vi "alignObjects.vi"(6 "alignment":T1, 8 "error in (no error)":errorcluster, 11 "GObjectsIn":refnum<class "GObject.lvclass">[](array[class])) -> (0 "error out":errorcluster, 3 "GObjectsOut":refnum<class "GObject.lvclass">[](array[class]))   [LabVIEW 2023, in "TLC_Scripto.lvlib"]
uses:
  TLC_Scripto.lvlib
  GObject/GObject.lvclass
  Ctrls/alignment.ctl
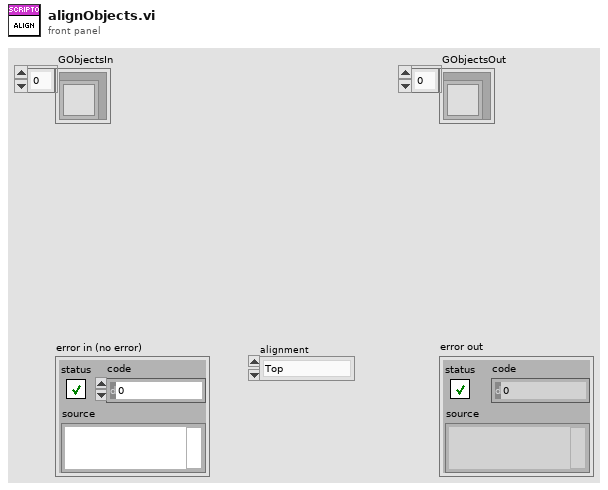
[diagram p1: front panel]
types:
  T1 = typedef "TLC_Scripto.lvlib/alignment.ctl" = enum16{"Top", "Bottom", "Left", "Right", "Center"}
  T2 = typedef "TLC_Scripto.lvlib/rectangle.ctl" = cluster{"left":i32, "top":i32, "right":i32, "bottom":i32}
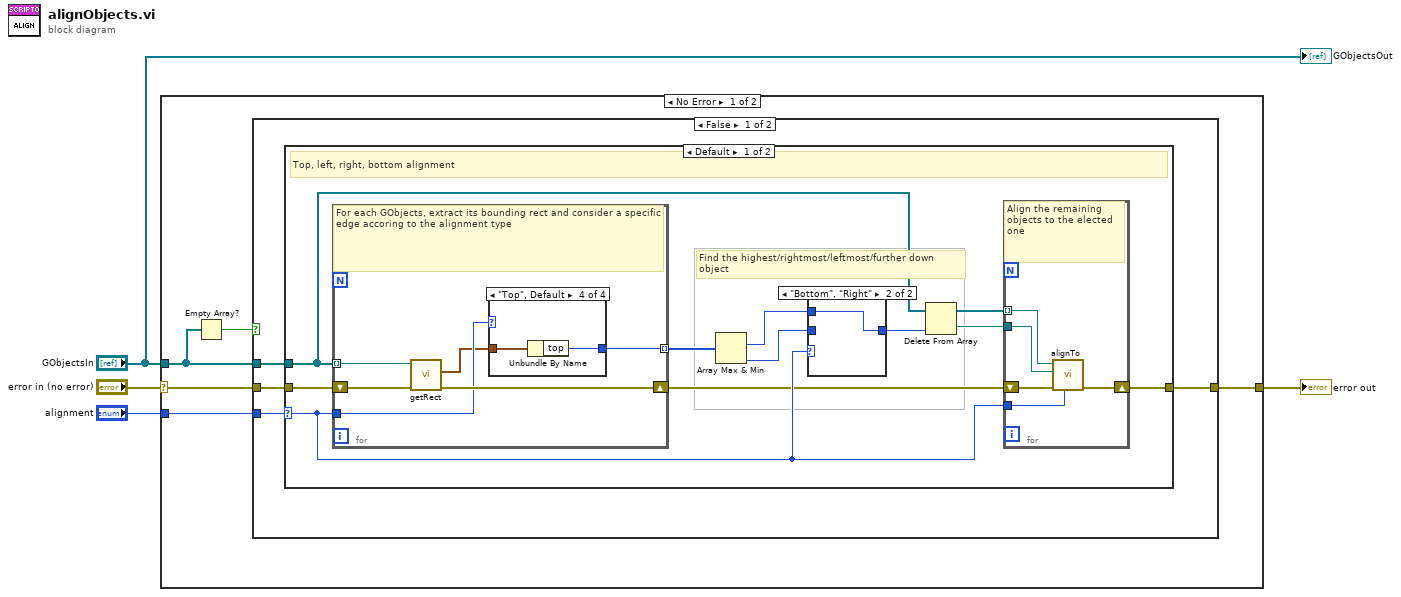
[diagram p0: block diagram]
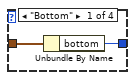
[diagram p3: hidden frame]
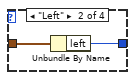
[diagram p4: hidden frame]
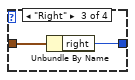
[diagram p5: hidden frame]
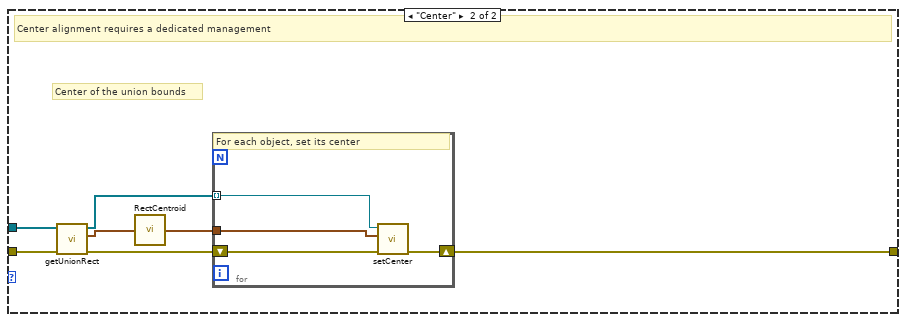
[diagram p6: hidden frame]
diagram:
  n1 = case shown="No Error" "error in (no error)" {
    selector: "error in (no error)" -> [w9 w58]
    tunnel: "GObjectsIn" -> [w7 _]
    tunnel: [w8 w58] -> w3
    tunnel: "alignment" -> [w5 _]
    frame No Error {
      n2 = Empty Array?(array=w7) -> (empty?=w6:bool)
      n3 = case shown="False" w6 {
        tunnel: w9 -> [w11 w57]
        tunnel: [w13 w57] -> w8
        tunnel: w7 -> [w12 _]
        tunnel: w5 -> [w10 _]
        frame False {
          n4 = case shown="Default" w10 {
            selector: w10 -> [w16 _]
            tunnel: [w14 w52] -> w13
            tunnel: w12 -> [w20 w50]
            tunnel: w11 -> [w24 w48]
            frame Default {
              # "Find the highest/rightmost/leftmost/further down object"
              # "Top, left, right, bottom alignment"
              n5 = for {
                tunnel: w20 -> [w37] mode=indexing
                shift-right: [w35] -> w15
                shift-left: w24 -> [w36]
                tunnel: w16 -> [w34]
                tunnel: [w32] -> w23 mode=indexing
                # "For each GObjects, extract its bounding rect and consider a specific edge accoring to the alignment type"
                n6 = call-dynamic "getRect.vi"("error in (no error)"=w36, "GObject in"=w37) -> ("error out"=w35:errorcluster, "rectangle"=w33:T2)  [unwired: 7 in, 1 out]
                n7 = case shown="\"Top\", Default" w34 {
                  tunnel: w33 -> [w39 w41 w43 w45]
                  tunnel: [w38 w40 w42 w44] -> w32
                  frame "Bottom" {
                    n8 = Unbundle By Name(w39) -> ("bottom"=w38:i32)
                  }
                  frame "Left" {
                    n9 = Unbundle By Name(w41) -> ("left"=w40:i32)
                  }
                  frame "Right" {
                    n10 = Unbundle By Name(w43) -> ("right"=w42:i32)
                  }
                  frame "Top", Default {
                    n11 = Unbundle By Name(w45) -> ("top"=w44:i32)
                  }
                }
              }
              n12 = Array Max & Min(array=w23) -> (max index (indices)=w21:i32, min index (indices)=w22:i32)  [unwired: 2 out]
              n13 = case shown="\"Bottom\", \"Right\"" w16 {
                tunnel: w22 -> [w30 _]
                tunnel: [w30 w31] -> w19
                tunnel: w21 -> [_ w31]
                frame "Top", "Left", Default {
                }
                frame "Bottom", "Right" {
                }
              }
              n14 = Delete From Array(array=w20, index=w19) -> (deleted portion=w18:refnum<class "GObject.lvclass">, array with subset deleted=w17:refnum<class "GObject.lvclass">[])  [unwired: 1 in]
              n15 = for {
                tunnel: w18 -> [w28]
                tunnel: w17 -> [w29] mode=indexing
                tunnel: w16 -> [w27]
                shift-right: [w25] -> w14
                shift-left: w15 -> [w26]
                # "Align the remaining objects to the elected one"
                n16 = call "alignTo.vi"("alignment"=w27, "error in (no error)"=w26, "targetObj"=w28, "GObject in"=w29) -> ("error out"=w25:errorcluster)  [unwired: 6 in, 1 out]
              }
            }
            frame "Center" {
              # "Center of the union bounds"
              # "Center alignment requires a dedicated management"
              n17 = call "getUnionRect.vi"("error in (no error)"=w48, "GObjects"=w50) -> ("error out"=w49:errorcluster, "unionRect"=w47:T2, "GObjects(dup)"=w51:refnum<class "GObject.lvclass">[])  [unwired: 7 in]
              n18 = call <vilib>:"RectCentroid.vi"("rect"=w47) -> ("point"=w46:cluster{"x":i16, "y":i16})
              n19 = for {
                tunnel: w51 -> [w56] mode=indexing
                shift-right: [w53] -> w52
                shift-left: w49 -> [w54]
                tunnel: w46 -> [w55]
                # "For each object, set its center"
                n20 = call-dynamic "setCenter.vi"("error in (no error)"=w54, "center"=w55, "GObject in"=w56) -> ("error out"=w53:errorcluster)  [unwired: 7 in, 1 out]
              }
            }
          }
        }
        frame True {
        }
      }
    }
    frame Error {
    }
  }
  "error out" <- w3
  "GObjectsOut" <- "GObjectsIn"
